vi "filtry.vi"() -> ()   [LabVIEW 2025]
uses:
  <vilib>/measure/macond.llb/IIR Filter for 1 Chan.vi
  <vilib>/measure/NI_MAPro.lvlib
  <vilib>/Analysis/NI_AALPro.lvlib
  <vilib>/measure/NI_MABase.lvlib
panel:
  in  "signal type 3":T1(ring)
  in  "phase 3":dbl format="%.2p"
  in  "amplitude 3":dbl=1.0 format="%0.2p"
  in  "frequency 3":dbl=10.0 format="%0.2p"
  in  "signal type 2":T1(ring)
  in  "phase 2":dbl format="%.2p"
  in  "amplitude 2":dbl=1.0 format="%0.2p"
  in  "frequency 2":dbl=10.0 format="%0.2p"
  out "przebieg czasowy":waveform(dbl)[](graph)
  in  "signal type":T1(ring)
  in  "phase":dbl format="%.2p"
  in  "amplitude":dbl=1.0 format="%0.2p"
  in  "frequency":dbl=10.0 format="%0.2p"
  out "widmo mocy":waveform(dbl)[](graph)
  out "charakterystyka skokowa filtra":waveform(dbl)[](graph)
  in  "stop":bool
  out "fazowa":cluster{"df":dbl, "df":dbl, "Phase H(w)":dbl[]}(graph)
  out "amplitudowa":cluster{"f0":dbl, "df":dbl, "Mag H(w)":dbl[]}(graph)
  in  "IIR filter specifications":T2={"Topology"=enum."Butterworth", "Type"=enum."Lowpass", "Order"=1, "Lower Fc"=100.0, "Upper Fc"=200.0, "PB Ripple"=1.0, "SB Attenuation"=60.0} {"PB Ripple" format="%0.2f"; "SB Attenuation" format="%0.2f"; "Lower Fc" format="%0.2p"; "Upper Fc" format="%0.2p"}
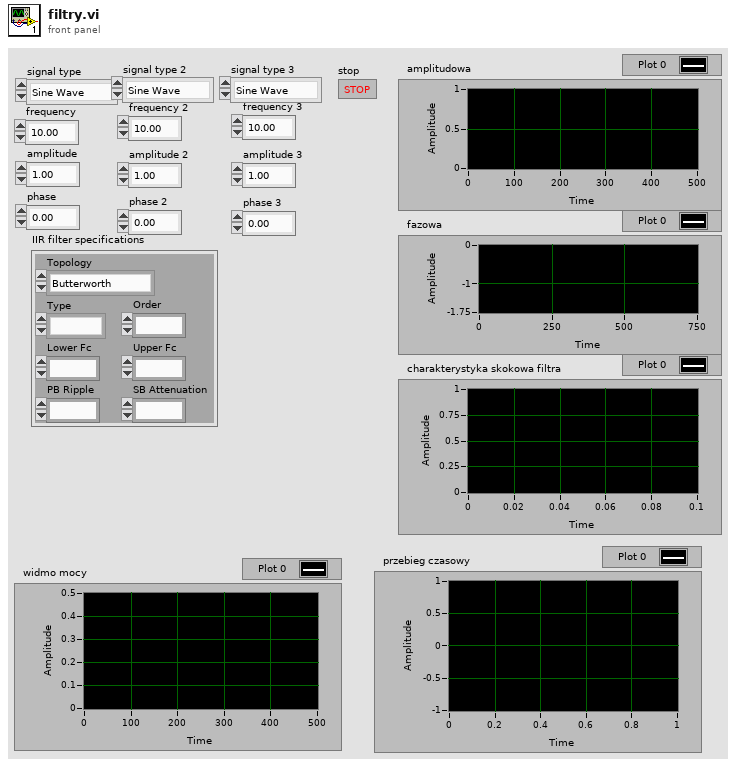
[diagram p1: front panel]
types:
  T1 = enum16{"Sine Wave", "Triangle Wave", "Square Wave", "Sawtooth Wave"}
  T2 = cluster{"Topology":enum16{"Off", "Butterworth", "Chebyshev", "Inverse Chebyshev", "Elliptic", "Bessel"}, "Type":enum16{"Lowpass", "Highpass", "Bandpass", "Bandstop"}, "Order":i32, "Lower Fc":dbl, "Upper Fc":dbl, "PB Ripple":dbl, "SB Attenuation":dbl}
  T3 = cluster{"magnitude H(w)":cluster{"f0":dbl, "df":dbl, "Mag H(w)":dbl[]}, "phase H(w)":cluster{"f0":dbl, "df":dbl, "Phase H(w)":dbl[]}, "order":i32}
  T4 = cluster{"df":dbl, "df":dbl, "Unwrapped Phase":dbl[]}
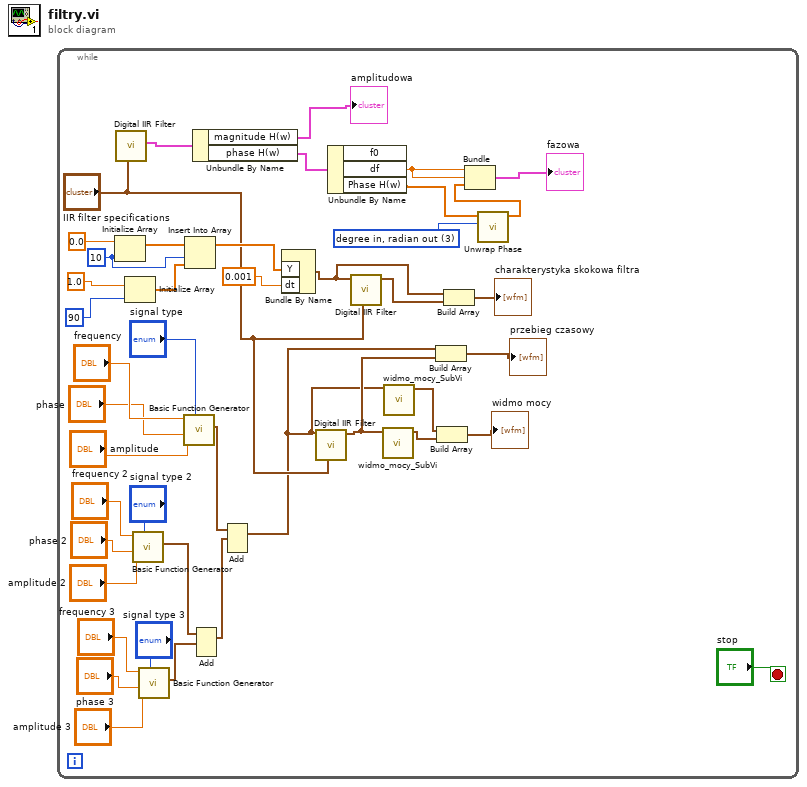
[diagram p0: block diagram]
diagram:
  n1 = while {
    stop <- "stop" stop-if-true
    w24 = 3 items=["radian in, radian out", "radian in, degree out", "degree in, degree out", "degree in, radian out"] ("phase unit")
    w31 = 10 ("dimension size")
    n2 = Initialize Array(0.0 ("element"), w31) -> (w33:dbl[])
    n3 = call-poly <vilib>:"Digital IIR Filter.vi"("IIR filter specifications"="IIR filter specifications") -> ("filter information"=w43:T3)  [unwired: 8 in, 2 out]
    n4 = Initialize Array(1.0 ("element"), 90 ("dimension size")) -> (w34:dbl[])
    n5 = call <vilib>:"Basic Function Generator.vi"("signal type"="signal type 2", "phase"="phase 2", "amplitude"="amplitude 2", "frequency"="frequency 2") -> ("signal out"=w5:waveform(dbl))  [unwired: 5 in, 2 out]
    n6 = call <vilib>:"Basic Function Generator.vi"("signal type"="signal type 3", "phase"="phase 3", "amplitude"="amplitude 3", "frequency"="frequency 3") -> ("signal out"=w4:waveform(dbl))  [unwired: 5 in, 2 out]
    n7 = call <vilib>:"Basic Function Generator.vi"("signal type"="signal type", "phase"="phase", "amplitude"="amplitude", "frequency"="frequency") -> ("signal out"=w3:waveform(dbl))  [unwired: 5 in, 2 out]
    n8 = Insert Into Array(array=w33, index=w31, new element=w34) -> (w35:dbl[])
    n9 = Add(1:w4, 2:w5) -> (0:w2:waveform(dbl))  [unwired: 1 in, 1 out]
    n10 = Unbundle By Name(w43) -> ("magnitude H(w)"=→"amplitudowa":cluster{"f0":dbl, "df":dbl, "Mag H(w)":dbl[]}, "phase H(w)"=w42:cluster{"f0":dbl, "df":dbl, "Phase H(w)":dbl[]})
    n11 = Add(1:w2, 2:w3) -> (0:w1:waveform(dbl))  [unwired: 1 in, 1 out]
    n12 = Bundle By Name("Y"=w35, "dt"=0.001) -> (w27:waveform(dbl))  [unwired: 1 in]
    n13 = call-poly <vilib>:"Digital IIR Filter.vi"("IIR filter specifications"="IIR filter specifications", "signal in"=w1) -> ("signal out"=w15:waveform(dbl))  [unwired: 7 in, 2 out]
    n14 = Unbundle By Name(w42) -> ("df"=w41:dbl, "Phase H(w)"=w40:dbl[])  [unwired: 1 out]
    n15 = call-poly <vilib>:"Digital IIR Filter.vi"("IIR filter specifications"="IIR filter specifications", "signal in"=w27) -> ("signal out"=w26:waveform(dbl))  [unwired: 7 in, 2 out]
    n16 = call "widmo_mocy_SubVi.vi"("signal in"=w15) -> ("widmo mocy"=w22:waveform(dbl))  [unwired: 10 in]
    n17 = call "widmo_mocy_SubVi.vi"("signal in"=w1) -> ("widmo mocy"=w23:waveform(dbl))  [unwired: 10 in]
    n18 = Build Array(w1, w15) -> (→"przebieg czasowy":waveform(dbl)[])
    n19 = Build Array(w23, w22) -> (→"widmo mocy":waveform(dbl)[])
    n20 = Build Array(w27, w26) -> (→"charakterystyka skokowa filtra":waveform(dbl)[])
    n21 = call <vilib>:"Unwrap Phase.vi"("phase unit"=w24, "Phase"=w40) -> ("Unwrapped Phase"=w37:dbl[])  [unwired: 8 in, 1 out]
    n22 = Bundle("df"=w41, "df"=w41, "Unwrapped Phase"=w37) -> (→"fazowa":T4)  [unwired: 1 in]
  }
